vi "cmc_Factorial Function.vi"() -> ()   [LabVIEW 2010]
panel:
  out "Factorial n! =":u64
  in  "Enter a positive integer n:":u64
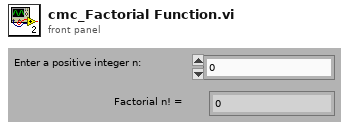
[diagram p1: front panel]
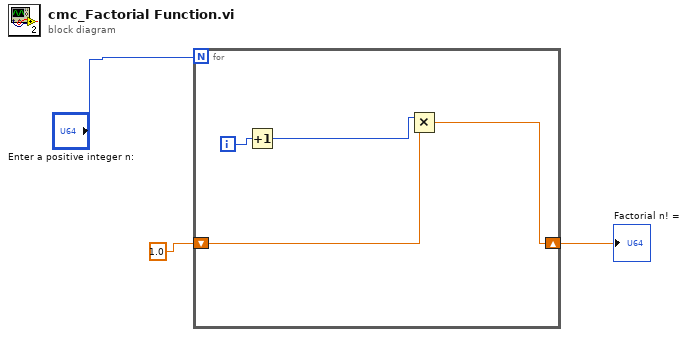
[diagram p0: block diagram]
diagram:
  n1 = for {
    N: "Enter a positive integer n:" -> [_]
    shift-right: [w4] -> w2
    shift-left: 1.0 -> [w5]
    i -> [w7]
    n2 = Increment(x=w7) -> (x+1=w6:i32)
    n3 = Multiply(x=w6, y=w5) -> (x*y=w4:dbl)
  }
  "Factorial n! =" <- w2
